vi "Get PS Status.vi"(8 "error in (no error)":errorcluster, 10 "Status":variant, 11 "PS Driver.lvlib:PS Driver.lvclass":refnum<class "PS Driver.lvclass">) -> (0 "error out":errorcluster, 2 "Status out":variant, 3 "PS Driver.lvlib:PS Driver.lvclass out":refnum<class "PS Driver.lvclass">)   [LabVIEW 2025, in "PS Driver.lvlib" / "PS Driver.lvclass"]
doc: "Author: Scott Hannahs <sth@magnet.fsu.edu>\n\nThis software is licensed for use under the “MIT License\"\nCopyright (c) 2025 Scott Hannahs, sth@sth@magnet.sthnet.net\n\nPermission is hereby granted, free of charge, to any person obtaining a copy of this software and associated documentation files (the \"Software\"), to deal in the Software without restriction, including without limitation the rights to use, copy, modify, merge, publish, distribute, sublicense, and/or sell copies of the Software, and to permit persons to whom the Software is furnished to do so, subject to the following conditions: The above copyright notice and this permission notice shall be included in all copies or substantial portions of the Software.\n\nTHE SOFTWARE IS PROVIDED \"AS IS\", WITHOUT WARRANTY OF ANY KIND, EXPRESS OR IMPLIED, INCLUDING BUT NOT LIMITED TO THE WARRANTIES OF MERCHANTABILITY, FITNESS FOR A PARTICULAR PURPOSE AND NONINFRINGEMENT. IN NO EVENT SHALL THE AUTHORS OR COPYRIGHT HOLDERS BE LIABLE FOR ANY CLAIM, DAMAGES OR OTHER LIABILITY, WHETHER IN AN ACTION OF CONTRACT, TORT OR OTHERWISE, ARISING FROM, OUT OF OR IN CONNECTION WITH THE SOFTWARE OR THE USE OR OTHER DEALINGS IN THE SOFTWARE."
uses:
  PS Driver.lvclass
  PS Driver.lvclass/PS Driver.ctl
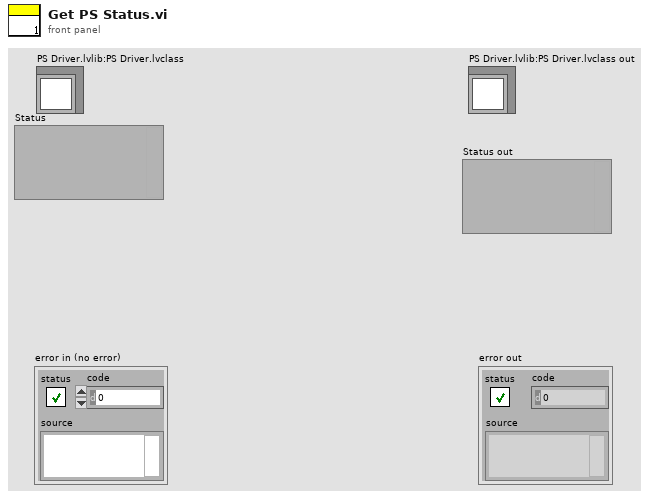
[diagram p1: front panel]
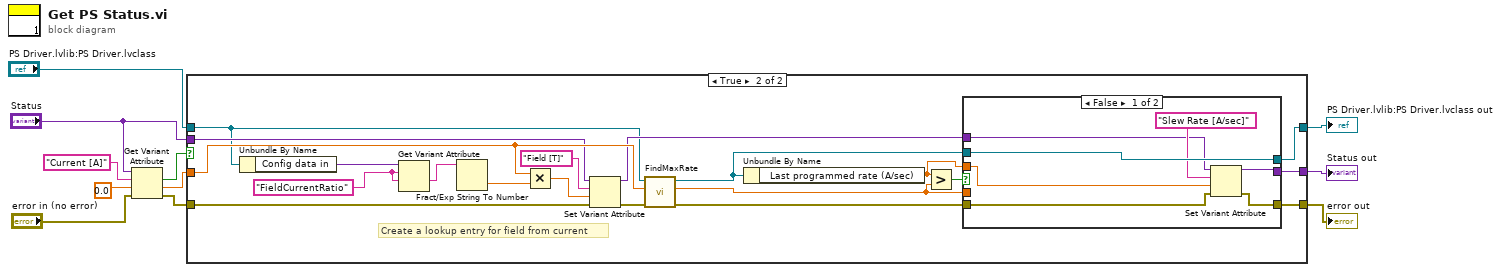
[diagram p0: block diagram]
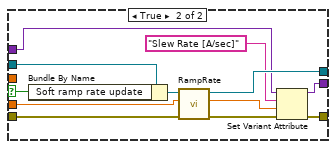
[diagram p3: hidden frame]
diagram:
  n1 = Get Variant Attribute(Variant="Status", name="Current [A]", default value (empty Variant)=0.0, error in="error in (no error)") -> (found=w9:bool, value=w8:dbl, error out=w5:errorcluster)  [unwired: 1 out]
  n2 = case shown="True" w9 {
    tunnel: w8 -> [_ w27]
    tunnel: "PS Driver.lvlib:PS Driver.lvclass" -> [w14 w20]
    tunnel: [w13 w30] -> w6
    tunnel: w5 -> [w13 w21]
    tunnel: [w14 w29] -> w4
    tunnel: "Status" -> [w12 w25]
    tunnel: [w12 w28] -> w2
    frame False {
    }
    frame True {
      w17 = "FieldCurrentRatio" ("name")
      # "Create a lookup entry for field from current"
      n3 = Unbundle By Name(w20) -> ("Config data in"=w18:variant)
      n4 = Get Variant Attribute(Variant=w18, name=w17, default value (empty Variant)=w17) -> (value=w19:string)  [unwired: 1 in, 3 out]
      n5 = Fract/Exp String To Number(string=w19) -> (number=w16:dbl)  [unwired: 3 in, 1 out]
      n6 = Multiply(x=w27, y=w16) -> (x*y=w23:dbl)
      n7 = Set Variant Attribute(Variant=w25, name="Field [T]", value=w23, error in=w21) -> (Variant out=w26:variant, error out=w22:errorcluster)  [unwired: 1 out]
      n8 = call "FindMaxRate.vi"("error in (no error)"=w22, "Current (A)"=w27, "PS Driver in"=w20) -> ("error out"=w31:errorcluster, "Max rate (A/sec)"=w32:dbl, "PS Driver out"=w33:refnum<class "PS Driver.lvclass">)  [unwired: 6 in]
      n9 = Unbundle By Name(w33) -> ("Last programmed rate (A/sec)"=w15:dbl)
      n10 = Greater?(x=w15, y=w32) -> (0:w34:bool)
      n11 = case shown="False" w34 {
        selector: w34 -> [_ w52]
        tunnel: w33 -> [w41 w53]
        tunnel: w32 -> [_ w51]
        tunnel: w31 -> [w36 w50]
        tunnel: [w37 w44] -> w30
        tunnel: [w41 w48] -> w29
        tunnel: w26 -> [w39 w47]
        tunnel: [w38 w43] -> w28
        tunnel: w15 -> [w35 _]
        frame False {
          n12 = Set Variant Attribute(Variant=w39, name="Slew Rate [A/sec]", value=w35, error in=w36) -> (Variant out=w38:variant, error out=w37:errorcluster)  [unwired: 1 out]
        }
        frame True {
          n13 = Bundle By Name(cluster=w53, "Soft ramp rate update"=w52) -> (w49:refnum<class "PS Driver.lvclass">)
          n14 = call-dynamic "RampRate.vi"("error in (no error)"=w50, "Ramp rate (A/sec)"=w51, "PS Driver in"=w49) -> ("error out"=w45:errorcluster, "Ramp rate out (A/s)"=w42:dbl, "PS Driver out"=w48:refnum<class "PS Driver.lvclass">)  [unwired: 6 in]
          n15 = Set Variant Attribute(Variant=w47, name="Slew Rate [A/sec]", value=w42, error in=w45) -> (Variant out=w43:variant, error out=w44:errorcluster)  [unwired: 1 out]
        }
      }
    }
  }
  "error out" <- w6
  "PS Driver.lvlib:PS Driver.lvclass out" <- w4
  "Status out" <- w2
